vi "adapter_pv.vi"(10 "configuration_pv":T1={"chunk"=4096, "mode"=1, "_reserved_0"=0, "width"=1920, "height"=1080, "framerate"=30, "divisor"=1, "profile"=3, "level"=255, "_reserved_1"=2, "bitrate"=0, "options_size"=-1, "options_data"=0, "_reserved_2"=0}, 11 "path in":path=path "hl2ss_ulm.dll") -> (2 "configuration":u64, 3 "path out":path)   [LabVIEW 2023]
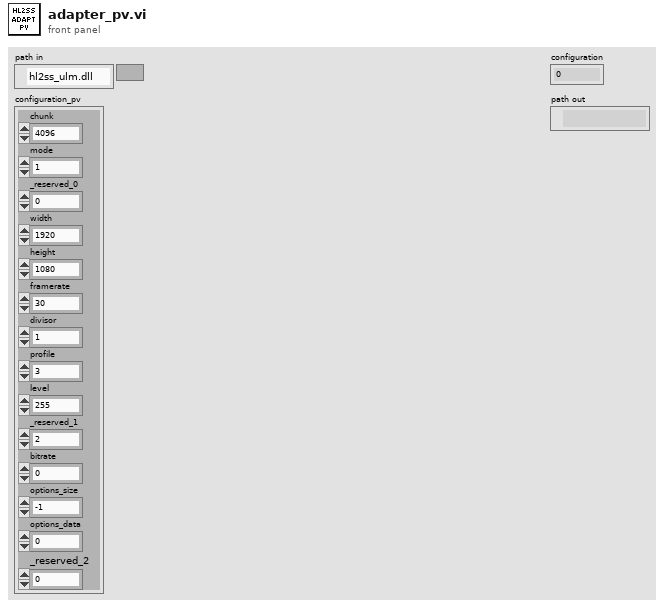
[diagram p1: front panel]
types:
  T1 = cluster{"chunk":u64, "mode":u8, "_reserved_0":u8, "width":u16, "height":u16, "framerate":u8, "divisor":u8, "profile":u8, "level":u8, "_reserved_1":u16, "bitrate":u32, "options_size":i64, "options_data":u64, "_reserved_2":u64}
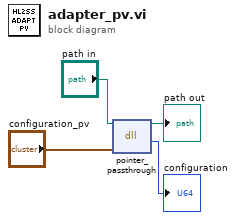
[diagram p0: block diagram]
diagram:
  n1 = dll-call lib="C:/Users/jcds/Documents/GitHub/hl2ss/extensions/client_labview/hl2ss_ulm.dll" fn="pointer_passthrough"(path in="path in", "p"="configuration_pv") -> (path out=→"path out":path, "return type"=→"configuration":u64)  [unwired: 3 in, 1 out]
